vi "BRAM U16_Xilinx.vi"(0 "Address 0":fxp<+,11,11>, 1 "Address0.Data":u16, 2 "Address0 Write?":bool, 3 "Address 1":fxp<+,11,11>, 4 "Address1.Data":u16, 5 "Address1 Write ?":bool) -> (15 "Address 0.Element Out":u16, 18 "Address 1.Element Out":u16)   [LabVIEW 2011]
uses:
  <vilib>/rvi/IPIntegrationNode/IPINode_Utilities/niFpgaIPINodeSimCore.vi
  <vilib>/rvi/XilinxIP/XIPIN_XNode/niFpgaXIPIN.xnode
  <userlib>/FPGA Library/Code Development/BRAM/Xilinx BRAM U16/Core/XilinxBRAMU16_492B662A4A00137524F1429F559EAF80.dll
  <vilib>/rvi/IPIntegrationNode/IPINode_Xnode/niFpgaIPINode.xnode
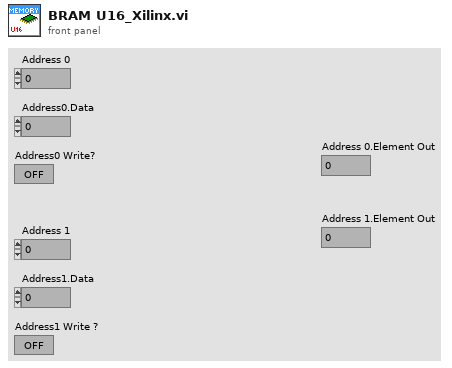
[diagram p1: front panel]
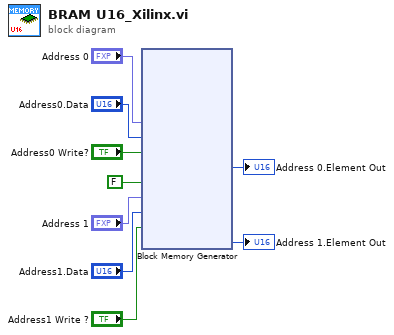
[diagram p0: block diagram]
diagram:
  n1 = xnode ("Block Memory Generator")("addra"="Address 0", "dina"="Address0.Data", "wea"="Address0 Write?", "clkb"=FALSE, "addrb"="Address 1", "dinb"="Address1.Data", "web"="Address1 Write ?") -> ("douta"=→"Address 0.Element Out":u16, "doutb"=→"Address 1.Element Out":u16)
